vi "BPF matlab.vi"   [LabVIEW 2014]
uses:
  <vilib>/imath/engines/lvmath2/RunTimeEngine/BuiltInFunctions/iir_cheby1ord/NIMS_iir_cheby1ord.vi
  <vilib>/imath/engines/lvmath2/RunTimeEngine/ErrorHandling/NIMS_Create Error From Enums.vi
  <vilib>/imath/engines/lvmath2/RunTimeEngine/BuiltInFunctions/iir_cheby1/NIMS_[2o]_iir_cheby1(I32,DBL,V).vi
  <vilib>/imath/engines/lvmath2/RunTimeEngine/BuiltInFunctions/freqzd/NIMS_freqzd().vi
  <vilib>/imathl/engines/lvmath/Functions/Error Handling/Create Error.vi
  <vilib>/imath/engines/lvmath2/RunTimeEngine/BuiltInFunctions/subplot/NIMS_subplot.vi
  <vilib>/imath/engines/lvmath2/RunTimeEngine/BuiltInFunctions/abs/NIMS_abs(signed).vi
  <instcachedir>/0/NIMS_abs(signed)_C4FCB8E6058B49B797C7C8D53CA5F6EC.lvgen/NIMS_abs(signed)_C4FCB8E6058B49B797C7C8D53CA5F6EC_006.vi
  <vilib>/imath/engines/lvmath2/RunTimeEngine/BuiltInFunctions/plot/NIMS_plot(RM, RM, Str).vi
  <vilib>/imath/engines/lvmath2/RunTimeEngine/ErrorHandling/NIMS_Finalize Error.vi
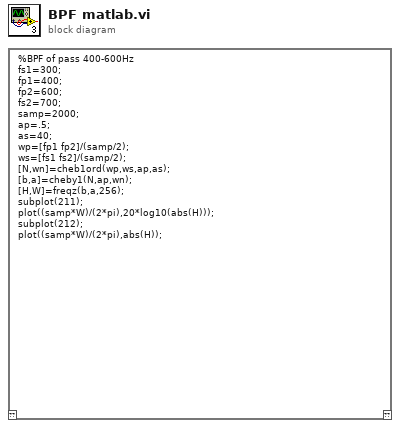
[diagram p0: block diagram]
diagram:
  n1 = mathscript code="%BPF of pass 400-600Hz\nfs1=300;\nfp1=400;\nfp2=600;\nfs2=700;\nsamp=2000;\nap=.5;\nas=40;\nwp=[fp1 fp2]/(samp/2);\nws=[fs1 fs2]/(samp/2);\n[N,wn]=cheb1ord(wp,ws,ap,as);\n[b,a]=cheby1(N,ap,wn);\n[H,W]=freqz(b,a,256);\nsubplot(211);\nplot((samp*W)/(2*pi),20*log10(abs(H)));\nsubplot(212);\nplot((samp*W)/(2*pi),abs(H));"() -> ()  [unwired: 1 in, 1 out]
